vi "GrayAnd2Values.vi"(8 "error in (no error)":errorcluster caption="错误输入（无错误）", 10 "阙值":u8=128, 11 "image data":T1 caption="图像数据") -> (0 "error out":errorcluster caption="错误输出", 3 "输出簇":T1)   [LabVIEW 2012]
uses:
  <vilib>/picture/picture.llb/imagedata.ctl
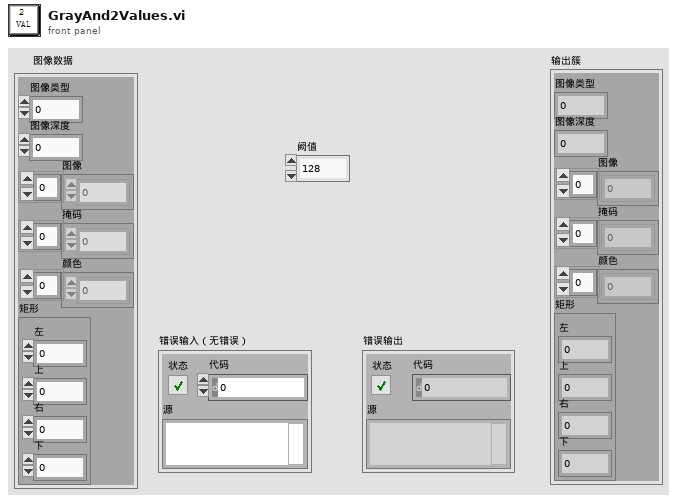
[diagram p1: front panel]
types:
  T1 = typedef "imagedata.ctl" = cluster{"image type":i32, "image depth":i32, "image":u8[], "mask":u8[], "colors":u32[], "Rectangle":cluster{"left":i16, "top":i16, "right":i16, "bottom":i16}}
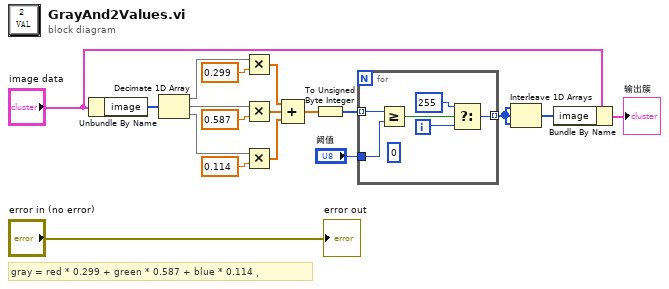
[diagram p0: block diagram]
diagram:
  # "gray = red * 0.299 + green * 0.587 + blue * 0.114，"
  n1 = Unbundle By Name("image data") -> ("image"=w18:u8[])
  n2 = Decimate 1D Array(w18) -> (w17:u8[], w15:u8[], w13:u8[])
  n3 = Multiply(x=w17, y=0.299) -> (x*y=w11:dbl[])
  n4 = Multiply(x=w15, y=0.587) -> (x*y=w10:dbl[])
  n5 = Multiply(x=w13, y=0.114) -> (x*y=w9:dbl[])
  n6 = Compound Arithmetic op=ADD(w11, w10, w9) -> (w8:dbl[])
  n7 = To Unsigned Byte Integer(number=w8) -> (unsigned 8bit integer=w3:u8[])
  n8 = for {
    tunnel: w3 -> [w22] mode=indexing
    tunnel: "阙值" -> [w21]
    tunnel: [w19] -> w1 mode=indexing
    i -> [w24]
    (unwired) 0 ("f")
    n9 = Greater Or Equal?(x=w22, y=w21) -> (x >= y?=w23:bool)
    n10 = Select(t=255, s=w23, f=w24) -> (s? t:f=w19:i32)
  }
  n11 = Interleave 1D Arrays(w1, w1, w1) -> (w4:i32[])
  n12 = Bundle By Name(cluster="image data", "image"=w4) -> (→"输出簇":T1)
  "error out" <- "error in (no error)"
